vi "Process Messages.vi"(8 "error in (no error)":errorcluster, 11 "Channel in":refnum<class "Channel.lvclass">) -> (0 "error out":errorcluster, 3 "Channel out":refnum<class "Channel.lvclass">)   [LabVIEW 2019, in "Channel.lvclass"]
uses:
  Channel.lvclass
  Channel.lvclass/Channel.ctl
  Libraries/Messaging/Messaging.lvlib
  Libraries/Audio Processing/Audio Processing.lvlib
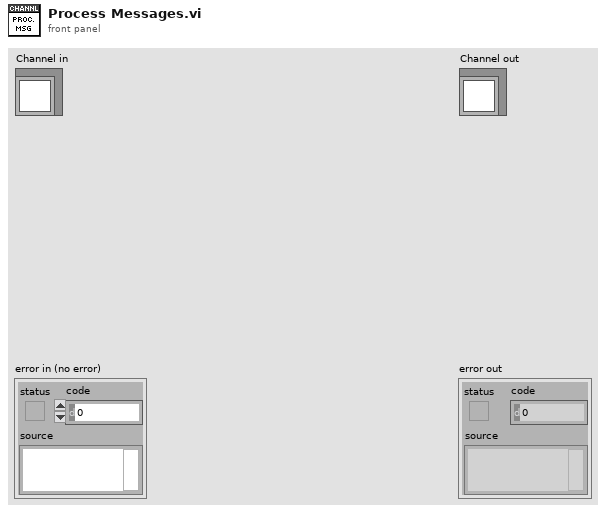
[diagram p1: front panel]
types:
  T1 = typedef "Messaging.lvlib/Message Cluster.ctl" = cluster{"Event":string, "Source":string, "Target":string, "Data":variant}
  T2 = typedef "Audio Processing.lvlib/Value Properties.ctl" = cluster{"Lower":dbl, "Upper":dbl, "Default":dbl, "Increment":dbl}
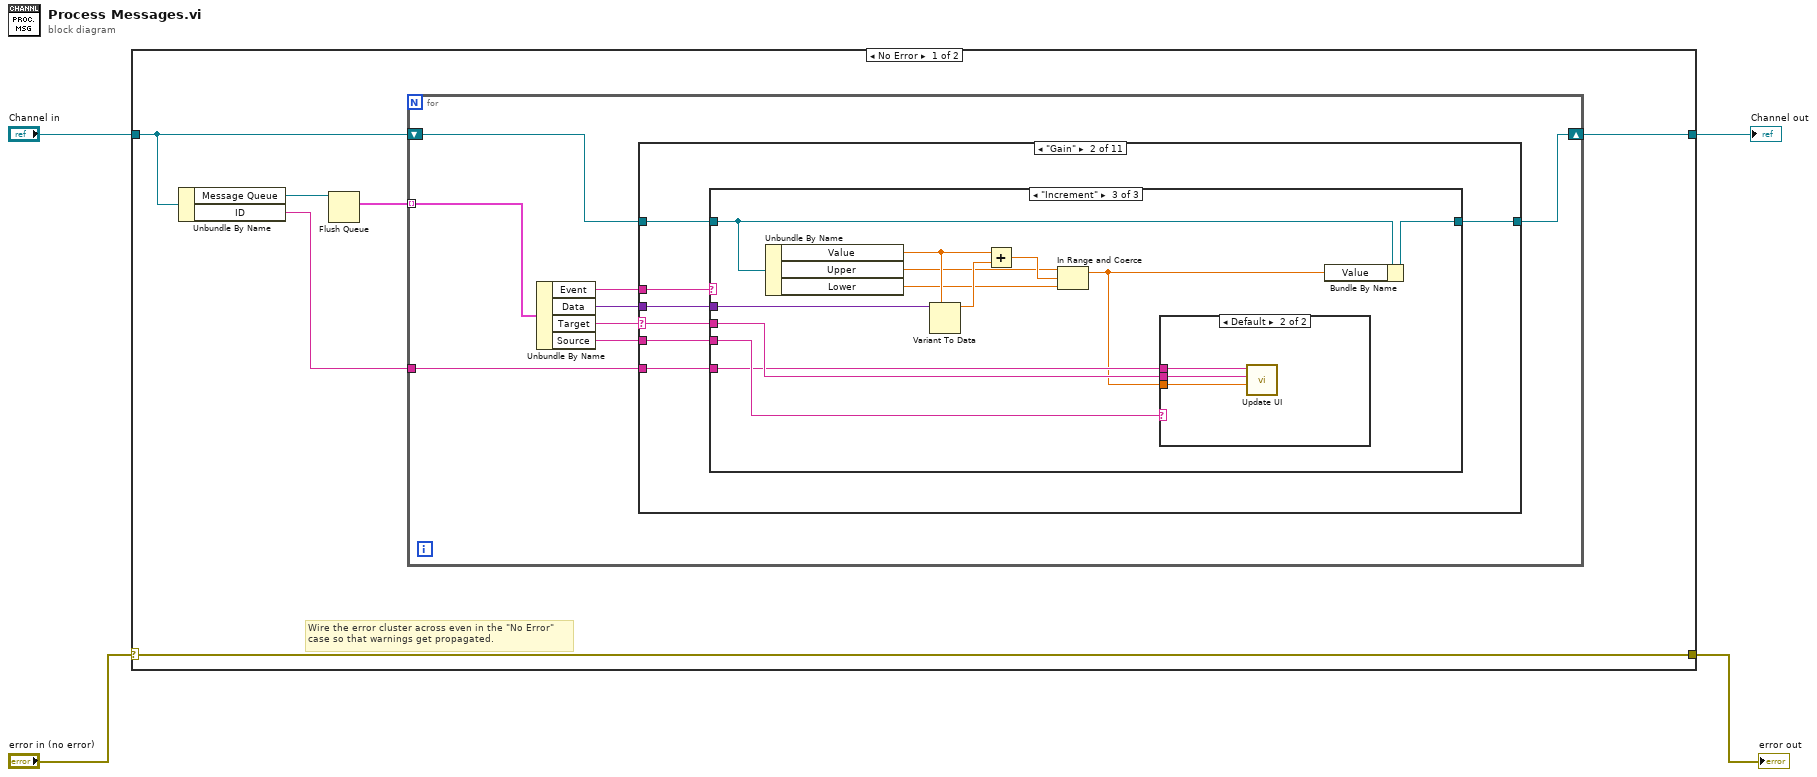
[diagram p0: block diagram]
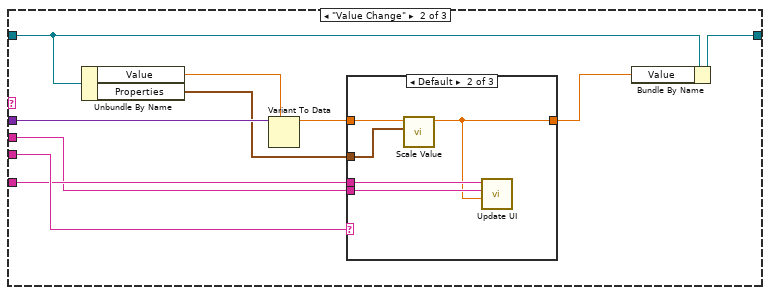
[diagram p4: hidden frame]
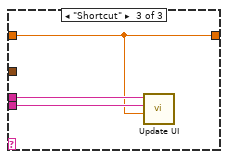
[diagram p6: hidden frame]
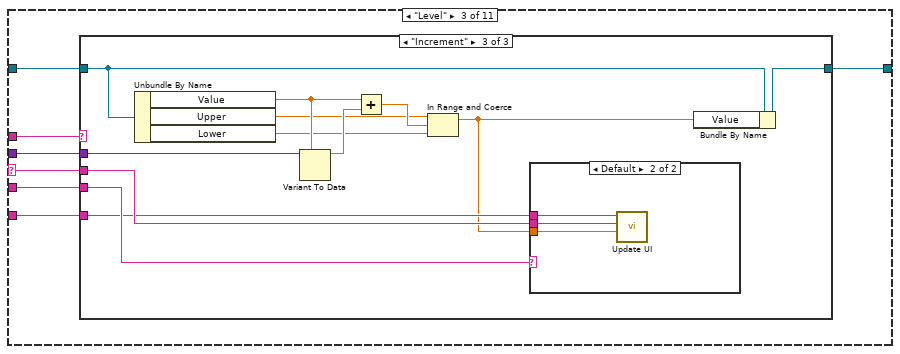
[diagram p8: hidden frame]
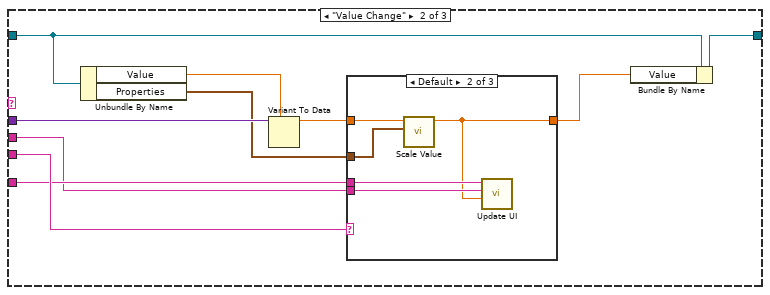
[diagram p10: hidden frame]
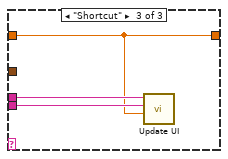
[diagram p12: hidden frame]
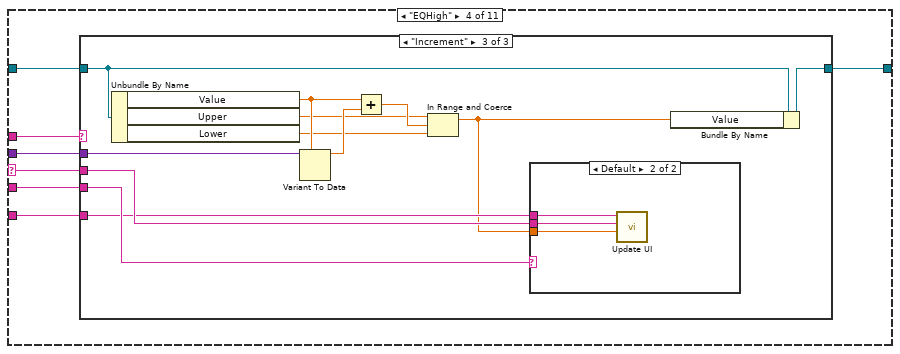
[diagram p14: hidden frame]
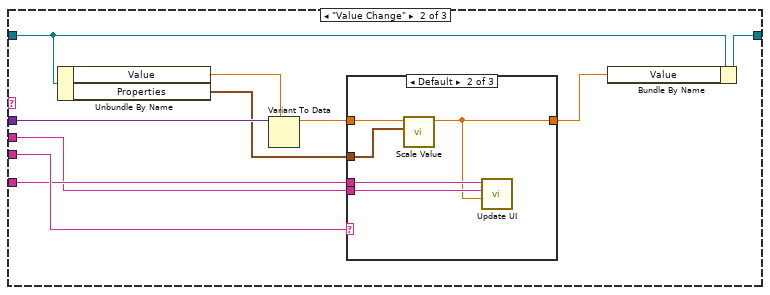
[diagram p16: hidden frame]
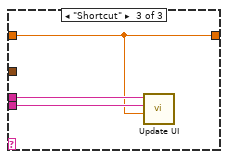
[diagram p18: hidden frame]
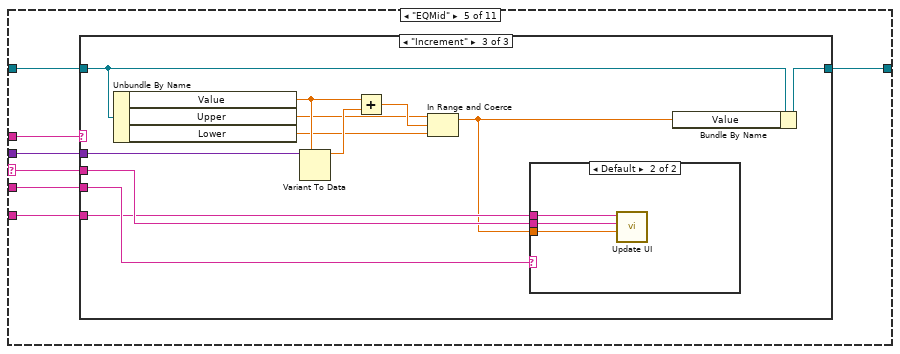
[diagram p20: hidden frame]
diagram:
  n1 = case shown="No Error" "error in (no error)" {
    selector: "error in (no error)" -> [w10 w389]
    tunnel: [w10 w389] -> w1
    tunnel: [w5 w388] -> w3
    tunnel: "Channel in" -> [w9 w388]
    frame No Error {
      # "Wire the error cluster across even in the \"No Error\"\ncase so that warnings get propagated."
      n2 = Unbundle By Name(w9) -> ("Message Queue"=w8:refnum<queue>, "ID"=w6:string)
      n3 = Flush Queue(queue=w8) -> (remaining elements=w7:T1[])  [unwired: 1 in, 2 out]
      n4 = for {
        shift-right: [w16] -> w5
        shift-left: w9 -> [w15]
        tunnel: w7 -> [w18] mode=indexing
        tunnel: w6 -> [w12]
        n5 = Unbundle By Name(w18) -> ("Event"=w14:string, "Data"=w13:variant, "Target"=w17:string, "Source"=w11:string)
        n6 = case shown="\"Gain\"" w17 {
          selector: w17 -> [_ w23 w65 w107 w148 w190 w232 w273 w302 w331 w360]
          tunnel: [w19 w20 w62 w104 w152 w194 w236 w275 w304 w333 w362] -> w16
          tunnel: w15 -> [w19 w26 w68 w110 w151 w193 w235 w276 w305 w334 w363]
          tunnel: w14 -> [_ w25 w67 w109 w150 w192 w234 w278 w307 w336 w365]
          tunnel: w13 -> [_ w24 w66 w108 w149 w191 w233 w277 w306 w335 w364]
          tunnel: w12 -> [_ w21 w63 w105 w146 w188 w230 w274 w303 w332 w361]
          tunnel: w11 -> [_ w22 w64 w106 w147 w189 w231 w272 w301 w330 w359]
          frame Default {
          }
          frame "Gain" {
            n7 = case shown="\"Increment\"" w25 {
              tunnel: [w27 w34 w56] -> w20
              tunnel: w26 -> [w27 w35 w57]
              tunnel: w24 -> [_ w36 w58]
              tunnel: w22 -> [_ w32 w55]
              tunnel: w23 -> [_ w30 w54]
              tunnel: w21 -> [_ w31 w53]
              frame Default {
              }
              frame "Value Change" {
                n8 = Unbundle By Name(w35) -> ("Value"=w37:dbl, "Properties"=w28:T2)
                n9 = Variant To Data(type=w37, Variant=w36) -> (data=w33:dbl)  [unwired: 1 in, 1 out]
                n10 = case shown="Default" w32 {
                  tunnel: w33 -> [w38 w41 w44]
                  tunnel: w30 -> [_ w43 w46]
                  tunnel: w31 -> [_ w42 w45]
                  tunnel: [w38 w39 w44] -> w29
                  tunnel: w28 -> [_ w40 _]
                  frame "UI" {
                  }
                  frame Default {
                    n11 = call "Scale Value.vi"("Limits"=w40, "Value"=w41) -> ("Scaled Value"=w39:dbl)  [unwired: 9 in]
                    n12 = call "Update UI.vi"("Data"=w39, "Target"=w43, "ID"=w42) -> ()  [unwired: 8 in, 1 out]
                  }
                  frame "Shortcut" {
                    n13 = call "Update UI.vi"("Data"=w44, "Target"=w46, "ID"=w45) -> ()  [unwired: 8 in, 1 out]
                  }
                }
                n14 = Bundle By Name(cluster=w35, "Value"=w29) -> (w34:refnum<class "Channel.lvclass">)
              }
              frame "Increment" {
                n15 = Unbundle By Name(w57) -> ("Value"=w52:dbl, "Upper"=w49:dbl, "Lower"=w48:dbl)
                n16 = Variant To Data(type=w52, Variant=w58) -> (data=w51:dbl)  [unwired: 1 in, 1 out]
                n17 = Add(x=w52, y=w51) -> (x+y=w50:dbl)
                n18 = In Range and Coerce(upper limit=w49, x=w50, lower limit=w48) -> (coerced(x)=w47:dbl)  [unwired: 1 out]
                n19 = case shown="Default" w55 {
                  tunnel: w47 -> [_ w61]
                  tunnel: w54 -> [_ w60]
                  tunnel: w53 -> [_ w59]
                  frame "UI" {
                  }
                  frame Default {
                    n20 = call "Update UI.vi"("Data"=w61, "Target"=w60, "ID"=w59) -> ()  [unwired: 8 in, 1 out]
                  }
                }
                n21 = Bundle By Name(cluster=w57, "Value"=w47) -> (w56:refnum<class "Channel.lvclass">)
              }
            }
          }
          frame "Level" {
            n22 = case shown="\"Increment\"" w67 {
              tunnel: [w69 w76 w98] -> w62
              tunnel: w68 -> [w69 w77 w99]
              tunnel: w66 -> [_ w78 w100]
              tunnel: w64 -> [_ w74 w97]
              tunnel: w65 -> [_ w72 w96]
              tunnel: w63 -> [_ w73 w95]
              frame Default {
              }
              frame "Value Change" {
                n23 = Unbundle By Name(w77) -> ("Value"=w79:dbl, "Properties"=w70:T2)
                n24 = Variant To Data(type=w79, Variant=w78) -> (data=w75:dbl)  [unwired: 1 in, 1 out]
                n25 = case shown="Default" w74 {
                  tunnel: w75 -> [w80 w83 w86]
                  tunnel: w72 -> [_ w85 w88]
                  tunnel: w73 -> [_ w84 w87]
                  tunnel: [w80 w81 w86] -> w71
                  tunnel: w70 -> [_ w82 _]
                  frame "UI" {
                  }
                  frame Default {
                    n26 = call "Scale Value.vi"("Limits"=w82, "Value"=w83) -> ("Scaled Value"=w81:dbl)  [unwired: 9 in]
                    n27 = call "Update UI.vi"("Data"=w81, "Target"=w85, "ID"=w84) -> ()  [unwired: 8 in, 1 out]
                  }
                  frame "Shortcut" {
                    n28 = call "Update UI.vi"("Data"=w86, "Target"=w88, "ID"=w87) -> ()  [unwired: 8 in, 1 out]
                  }
                }
                n29 = Bundle By Name(cluster=w77, "Value"=w71) -> (w76:refnum<class "Channel.lvclass">)
              }
              frame "Increment" {
                n30 = Unbundle By Name(w99) -> ("Value"=w94:dbl, "Upper"=w91:dbl, "Lower"=w90:dbl)
                n31 = Variant To Data(type=w94, Variant=w100) -> (data=w93:dbl)  [unwired: 1 in, 1 out]
                n32 = Add(x=w94, y=w93) -> (x+y=w92:dbl)
                n33 = In Range and Coerce(upper limit=w91, x=w92, lower limit=w90) -> (coerced(x)=w89:dbl)  [unwired: 1 out]
                n34 = case shown="Default" w97 {
                  tunnel: w89 -> [_ w103]
                  tunnel: w96 -> [_ w102]
                  tunnel: w95 -> [_ w101]
                  frame "UI" {
                  }
                  frame Default {
                    n35 = call "Update UI.vi"("Data"=w103, "Target"=w102, "ID"=w101) -> ()  [unwired: 8 in, 1 out]
                  }
                }
                n36 = Bundle By Name(cluster=w99, "Value"=w89) -> (w98:refnum<class "Channel.lvclass">)
              }
            }
          }
          frame "EQHigh" {
            n37 = case shown="\"Increment\"" w109 {
              tunnel: [w111 w118 w140] -> w104
              tunnel: w110 -> [w111 w119 w141]
              tunnel: w108 -> [_ w120 w142]
              tunnel: w106 -> [_ w116 w139]
              tunnel: w107 -> [_ w114 w138]
              tunnel: w105 -> [_ w115 w137]
              frame Default {
              }
              frame "Value Change" {
                n38 = Unbundle By Name(w119) -> ("Value"=w121:dbl, "Properties"=w112:T2)
                n39 = Variant To Data(type=w121, Variant=w120) -> (data=w117:dbl)  [unwired: 1 in, 1 out]
                n40 = case shown="Default" w116 {
                  tunnel: w117 -> [w122 w125 w128]
                  tunnel: w114 -> [_ w127 w130]
                  tunnel: w115 -> [_ w126 w129]
                  tunnel: [w122 w123 w128] -> w113
                  tunnel: w112 -> [_ w124 _]
                  frame "UI" {
                  }
                  frame Default {
                    n41 = call "Scale Value.vi"("Limits"=w124, "Value"=w125) -> ("Scaled Value"=w123:dbl)  [unwired: 9 in]
                    n42 = call "Update UI.vi"("Data"=w123, "Target"=w127, "ID"=w126) -> ()  [unwired: 8 in, 1 out]
                  }
                  frame "Shortcut" {
                    n43 = call "Update UI.vi"("Data"=w128, "Target"=w130, "ID"=w129) -> ()  [unwired: 8 in, 1 out]
                  }
                }
                n44 = Bundle By Name(cluster=w119, "Value"=w113) -> (w118:refnum<class "Channel.lvclass">)
              }
              frame "Increment" {
                n45 = Unbundle By Name(w141) -> ("Value"=w136:dbl, "Upper"=w133:dbl, "Lower"=w132:dbl)
                n46 = Variant To Data(type=w136, Variant=w142) -> (data=w135:dbl)  [unwired: 1 in, 1 out]
                n47 = Add(x=w136, y=w135) -> (x+y=w134:dbl)
                n48 = In Range and Coerce(upper limit=w133, x=w134, lower limit=w132) -> (coerced(x)=w131:dbl)  [unwired: 1 out]
                n49 = case shown="Default" w139 {
                  tunnel: w131 -> [_ w145]
                  tunnel: w138 -> [_ w144]
                  tunnel: w137 -> [_ w143]
                  frame "UI" {
                  }
                  frame Default {
                    n50 = call "Update UI.vi"("Data"=w145, "Target"=w144, "ID"=w143) -> ()  [unwired: 8 in, 1 out]
                  }
                }
                n51 = Bundle By Name(cluster=w141, "Value"=w131) -> (w140:refnum<class "Channel.lvclass">)
              }
            }
          }
          frame "EQMid" {
            n52 = case shown="\"Increment\"" w150 {
              tunnel: [w153 w160 w182] -> w152
              tunnel: w151 -> [w153 w161 w183]
              tunnel: w149 -> [_ w162 w184]
              tunnel: w147 -> [_ w158 w181]
              tunnel: w148 -> [_ w156 w180]
              tunnel: w146 -> [_ w157 w179]
              frame Default {
              }
              frame "Value Change" {
                n53 = Unbundle By Name(w161) -> ("Value"=w163:dbl, "Properties"=w154:T2)
                n54 = Variant To Data(type=w163, Variant=w162) -> (data=w159:dbl)  [unwired: 1 in, 1 out]
                n55 = case shown="Default" w158 {
                  tunnel: w159 -> [w164 w167 w170]
                  tunnel: w156 -> [_ w169 w172]
                  tunnel: w157 -> [_ w168 w171]
                  tunnel: [w164 w165 w170] -> w155
                  tunnel: w154 -> [_ w166 _]
                  frame "UI" {
                  }
                  frame Default {
                    n56 = call "Scale Value.vi"("Limits"=w166, "Value"=w167) -> ("Scaled Value"=w165:dbl)  [unwired: 9 in]
                    n57 = call "Update UI.vi"("Data"=w165, "Target"=w169, "ID"=w168) -> ()  [unwired: 8 in, 1 out]
                  }
                  frame "Shortcut" {
                    n58 = call "Update UI.vi"("Data"=w170, "Target"=w172, "ID"=w171) -> ()  [unwired: 8 in, 1 out]
                  }
                }
                n59 = Bundle By Name(cluster=w161, "Value"=w155) -> (w160:refnum<class "Channel.lvclass">)
              }
              frame "Increment" {
                n60 = Unbundle By Name(w183) -> ("Value"=w178:dbl, "Upper"=w175:dbl, "Lower"=w174:dbl)
                n61 = Variant To Data(type=w178, Variant=w184) -> (data=w177:dbl)  [unwired: 1 in, 1 out]
                n62 = Add(x=w178, y=w177) -> (x+y=w176:dbl)
                n63 = In Range and Coerce(upper limit=w175, x=w176, lower limit=w174) -> (coerced(x)=w173:dbl)  [unwired: 1 out]
                n64 = case shown="Default" w181 {
                  tunnel: w173 -> [_ w187]
                  tunnel: w180 -> [_ w186]
                  tunnel: w179 -> [_ w185]
                  frame "UI" {
                  }
                  frame Default {
                    n65 = call "Update UI.vi"("Data"=w187, "Target"=w186, "ID"=w185) -> ()  [unwired: 8 in, 1 out]
                  }
                }
                n66 = Bundle By Name(cluster=w183, "Value"=w173) -> (w182:refnum<class "Channel.lvclass">)
              }
            }
          }
          frame "EQLow" {
            n67 = case shown="\"Increment\"" w192 {
              tunnel: [w195 w202 w224] -> w194
              tunnel: w193 -> [w195 w203 w225]
              tunnel: w191 -> [_ w204 w226]
              tunnel: w189 -> [_ w200 w223]
              tunnel: w190 -> [_ w198 w222]
              tunnel: w188 -> [_ w199 w221]
              frame Default {
              }
              frame "Value Change" {
                n68 = Unbundle By Name(w203) -> ("Value"=w205:dbl, "Properties"=w196:T2)
                n69 = Variant To Data(type=w205, Variant=w204) -> (data=w201:dbl)  [unwired: 1 in, 1 out]
                n70 = case shown="Default" w200 {
                  tunnel: w201 -> [w206 w209 w212]
                  tunnel: w198 -> [_ w211 w214]
                  tunnel: w199 -> [_ w210 w213]
                  tunnel: [w206 w207 w212] -> w197
                  tunnel: w196 -> [_ w208 _]
                  frame "UI" {
                  }
                  frame Default {
                    n71 = call "Scale Value.vi"("Limits"=w208, "Value"=w209) -> ("Scaled Value"=w207:dbl)  [unwired: 9 in]
                    n72 = call "Update UI.vi"("Data"=w207, "Target"=w211, "ID"=w210) -> ()  [unwired: 8 in, 1 out]
                  }
                  frame "Shortcut" {
                    n73 = call "Update UI.vi"("Data"=w212, "Target"=w214, "ID"=w213) -> ()  [unwired: 8 in, 1 out]
                  }
                }
                n74 = Bundle By Name(cluster=w203, "Value"=w197) -> (w202:refnum<class "Channel.lvclass">)
              }
              frame "Increment" {
                n75 = Unbundle By Name(w225) -> ("Value"=w220:dbl, "Upper"=w217:dbl, "Lower"=w216:dbl)
                n76 = Variant To Data(type=w220, Variant=w226) -> (data=w219:dbl)  [unwired: 1 in, 1 out]
                n77 = Add(x=w220, y=w219) -> (x+y=w218:dbl)
                n78 = In Range and Coerce(upper limit=w217, x=w218, lower limit=w216) -> (coerced(x)=w215:dbl)  [unwired: 1 out]
                n79 = case shown="Default" w223 {
                  tunnel: w215 -> [_ w229]
                  tunnel: w222 -> [_ w228]
                  tunnel: w221 -> [_ w227]
                  frame "UI" {
                  }
                  frame Default {
                    n80 = call "Update UI.vi"("Data"=w229, "Target"=w228, "ID"=w227) -> ()  [unwired: 8 in, 1 out]
                  }
                }
                n81 = Bundle By Name(cluster=w225, "Value"=w215) -> (w224:refnum<class "Channel.lvclass">)
              }
            }
          }
          frame "EQFilter" {
            n82 = case shown="\"Increment\"" w234 {
              tunnel: [w237 w244 w266] -> w236
              tunnel: w235 -> [w237 w245 w267]
              tunnel: w233 -> [_ w246 w268]
              tunnel: w231 -> [_ w242 w265]
              tunnel: w232 -> [_ w240 w264]
              tunnel: w230 -> [_ w241 w263]
              frame Default {
              }
              frame "Value Change" {
                n83 = Unbundle By Name(w245) -> ("Value"=w247:dbl, "Properties"=w238:T2)
                n84 = Variant To Data(type=w247, Variant=w246) -> (data=w243:dbl)  [unwired: 1 in, 1 out]
                n85 = case shown="Default" w242 {
                  tunnel: w243 -> [w248 w251 w254]
                  tunnel: w240 -> [_ w253 w256]
                  tunnel: w241 -> [_ w252 w255]
                  tunnel: [w248 w249 w254] -> w239
                  tunnel: w238 -> [_ w250 _]
                  frame "UI" {
                  }
                  frame Default {
                    n86 = call "Scale Value.vi"("Limits"=w250, "Value"=w251) -> ("Scaled Value"=w249:dbl)  [unwired: 9 in]
                    n87 = call "Update UI.vi"("Data"=w249, "Target"=w253, "ID"=w252) -> ()  [unwired: 8 in, 1 out]
                  }
                  frame "Shortcut" {
                    n88 = call "Update UI.vi"("Data"=w254, "Target"=w256, "ID"=w255) -> ()  [unwired: 8 in, 1 out]
                  }
                }
                n89 = Bundle By Name(cluster=w245, "Value"=w239) -> (w244:refnum<class "Channel.lvclass">)
              }
              frame "Increment" {
                n90 = Unbundle By Name(w267) -> ("Value"=w262:dbl, "Upper"=w259:dbl, "Lower"=w258:dbl)
                n91 = Variant To Data(type=w262, Variant=w268) -> (data=w261:dbl)  [unwired: 1 in, 1 out]
                n92 = Add(x=w262, y=w261) -> (x+y=w260:dbl)
                n93 = In Range and Coerce(upper limit=w259, x=w260, lower limit=w258) -> (coerced(x)=w257:dbl)  [unwired: 1 out]
                n94 = case shown="Default" w265 {
                  tunnel: w257 -> [_ w271]
                  tunnel: w264 -> [_ w270]
                  tunnel: w263 -> [_ w269]
                  frame "UI" {
                  }
                  frame Default {
                    n95 = call "Update UI.vi"("Data"=w271, "Target"=w270, "ID"=w269) -> ()  [unwired: 8 in, 1 out]
                  }
                }
                n96 = Bundle By Name(cluster=w267, "Value"=w257) -> (w266:refnum<class "Channel.lvclass">)
              }
            }
          }
          frame "EQHighKill" {
            n97 = case shown="\"Value Change\"" w278 {
              tunnel: w277 -> [_ w286 _]
              tunnel: w276 -> [w279 w285 w297]
              tunnel: [w279 w284 w296] -> w275
              tunnel: w274 -> [_ w282 w295]
              tunnel: w273 -> [_ w281 w294]
              tunnel: w272 -> [_ w280 w293]
              frame Default {
              }
              frame "Value Change" {
                n98 = Unbundle By Name(w285) -> ("Kill"=w287:bool)
                n99 = Variant To Data(type=w287, Variant=w286) -> (data=w283:bool)  [unwired: 1 in, 1 out]
                n100 = case shown="Default" w280 {
                  tunnel: w283 -> [_ w290]
                  tunnel: w281 -> [_ w289]
                  tunnel: w282 -> [_ w288]
                  frame "UI" {
                  }
                  frame Default {
                    n101 = call "Update UI.vi"("Data"=w290, "Target"=w289, "ID"=w288) -> ()  [unwired: 8 in, 1 out]
                  }
                }
                n102 = Bundle By Name(cluster=w285, "Kill"=w283) -> (w284:refnum<class "Channel.lvclass">)
              }
              frame "Toggle" {
                n103 = Unbundle By Name(w297) -> ("Kill"=w292:bool)
                n104 = Not(x=w292) -> (.not. x?=w291:bool)
                n105 = case shown="Default" w293 {
                  tunnel: w291 -> [_ w300]
                  tunnel: w294 -> [_ w299]
                  tunnel: w295 -> [_ w298]
                  frame "UI" {
                  }
                  frame Default {
                    n106 = call "Update UI.vi"("Data"=w300, "Target"=w299, "ID"=w298) -> ()  [unwired: 8 in, 1 out]
                  }
                }
                n107 = Bundle By Name(cluster=w297, "Kill"=w291) -> (w296:refnum<class "Channel.lvclass">)
              }
            }
          }
          frame "EQMidKill" {
            n108 = case shown="\"Value Change\"" w307 {
              tunnel: w306 -> [_ w315 _]
              tunnel: w305 -> [w308 w314 w326]
              tunnel: [w308 w313 w325] -> w304
              tunnel: w303 -> [_ w311 w324]
              tunnel: w302 -> [_ w310 w323]
              tunnel: w301 -> [_ w309 w322]
              frame Default {
              }
              frame "Value Change" {
                n109 = Unbundle By Name(w314) -> ("Kill"=w316:bool)
                n110 = Variant To Data(type=w316, Variant=w315) -> (data=w312:bool)  [unwired: 1 in, 1 out]
                n111 = case shown="Default" w309 {
                  tunnel: w312 -> [_ w319]
                  tunnel: w310 -> [_ w318]
                  tunnel: w311 -> [_ w317]
                  frame "UI" {
                  }
                  frame Default {
                    n112 = call "Update UI.vi"("Data"=w319, "Target"=w318, "ID"=w317) -> ()  [unwired: 8 in, 1 out]
                  }
                }
                n113 = Bundle By Name(cluster=w314, "Kill"=w312) -> (w313:refnum<class "Channel.lvclass">)
              }
              frame "Toggle" {
                n114 = Unbundle By Name(w326) -> ("Kill"=w321:bool)
                n115 = Not(x=w321) -> (.not. x?=w320:bool)
                n116 = case shown="Default" w322 {
                  tunnel: w320 -> [_ w329]
                  tunnel: w323 -> [_ w328]
                  tunnel: w324 -> [_ w327]
                  frame "UI" {
                  }
                  frame Default {
                    n117 = call "Update UI.vi"("Data"=w329, "Target"=w328, "ID"=w327) -> ()  [unwired: 8 in, 1 out]
                  }
                }
                n118 = Bundle By Name(cluster=w326, "Kill"=w320) -> (w325:refnum<class "Channel.lvclass">)
              }
            }
          }
          frame "EQLowKill" {
            n119 = case shown="\"Value Change\"" w336 {
              tunnel: w335 -> [_ w344 _]
              tunnel: w334 -> [w337 w343 w355]
              tunnel: [w337 w342 w354] -> w333
              tunnel: w332 -> [_ w340 w353]
              tunnel: w331 -> [_ w339 w352]
              tunnel: w330 -> [_ w338 w351]
              frame Default {
              }
              frame "Value Change" {
                n120 = Unbundle By Name(w343) -> ("Kill"=w345:bool)
                n121 = Variant To Data(type=w345, Variant=w344) -> (data=w341:bool)  [unwired: 1 in, 1 out]
                n122 = case shown="Default" w338 {
                  tunnel: w341 -> [_ w348]
                  tunnel: w339 -> [_ w347]
                  tunnel: w340 -> [_ w346]
                  frame "UI" {
                  }
                  frame Default {
                    n123 = call "Update UI.vi"("Data"=w348, "Target"=w347, "ID"=w346) -> ()  [unwired: 8 in, 1 out]
                  }
                }
                n124 = Bundle By Name(cluster=w343, "Kill"=w341) -> (w342:refnum<class "Channel.lvclass">)
              }
              frame "Toggle" {
                n125 = Unbundle By Name(w355) -> ("Kill"=w350:bool)
                n126 = Not(x=w350) -> (.not. x?=w349:bool)
                n127 = case shown="Default" w351 {
                  tunnel: w349 -> [_ w358]
                  tunnel: w352 -> [_ w357]
                  tunnel: w353 -> [_ w356]
                  frame "UI" {
                  }
                  frame Default {
                    n128 = call "Update UI.vi"("Data"=w358, "Target"=w357, "ID"=w356) -> ()  [unwired: 8 in, 1 out]
                  }
                }
                n129 = Bundle By Name(cluster=w355, "Kill"=w349) -> (w354:refnum<class "Channel.lvclass">)
              }
            }
          }
          frame "HeadphoneOutput" {
            n130 = case shown="\"Value Change\"" w365 {
              tunnel: w364 -> [_ w373 _]
              tunnel: w363 -> [w366 w372 w384]
              tunnel: [w366 w371 w383] -> w362
              tunnel: w361 -> [_ w369 w382]
              tunnel: w360 -> [_ w368 w381]
              tunnel: w359 -> [_ w367 w380]
              frame Default {
              }
              frame "Value Change" {
                n131 = Unbundle By Name(w372) -> ("HeadphoneOutput"=w374:bool)
                n132 = Variant To Data(type=w374, Variant=w373) -> (data=w370:bool)  [unwired: 1 in, 1 out]
                n133 = case shown="Default" w367 {
                  tunnel: w370 -> [_ w377]
                  tunnel: w368 -> [_ w376]
                  tunnel: w369 -> [_ w375]
                  frame "UI" {
                  }
                  frame Default {
                    n134 = call "Update UI.vi"("Data"=w377, "Target"=w376, "ID"=w375) -> ()  [unwired: 8 in, 1 out]
                  }
                }
                n135 = Bundle By Name(cluster=w372, "HeadphoneOutput"=w370) -> (w371:refnum<class "Channel.lvclass">)
              }
              frame "Toggle" {
                n136 = Unbundle By Name(w384) -> ("HeadphoneOutput"=w379:bool)
                n137 = Not(x=w379) -> (.not. x?=w378:bool)
                n138 = case shown="Default" w380 {
                  tunnel: w378 -> [_ w387]
                  tunnel: w381 -> [_ w386]
                  tunnel: w382 -> [_ w385]
                  frame "UI" {
                  }
                  frame Default {
                    n139 = call "Update UI.vi"("Data"=w387, "Target"=w386, "ID"=w385) -> ()  [unwired: 8 in, 1 out]
                  }
                }
                n140 = Bundle By Name(cluster=w384, "HeadphoneOutput"=w378) -> (w383:refnum<class "Channel.lvclass">)
              }
            }
          }
        }
      }
    }
    frame Error {
    }
  }
  "error out" <- w1
  "Channel out" <- w3
